vi "ElevShifter.vi"(5 "MaxPwr":dbl, 8 "Shift?":bool, 9 "PwrIn":dbl) -> (3 "PwrOut":dbl)   [LabVIEW 2017]
uses:
  <vilib>/Rock Robotics/WPI/Solenoid/Deprecated/WPI_SolenoidSetBool.vi
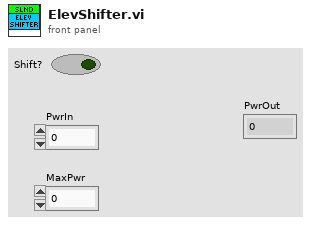
[diagram p1: front panel]
types:
  T1 = typedef "WPI_SolenoidDevRef.ctl" = cluster{"DevStatus":errorcluster, "Pneumatics Control Module":u8, "Forward Solenoid Channel":T2, "Reverse Solenoid Channel":T2}
  T2 = typedef "WPI_SolenoidChannel.ctl" = enum8{"Solenoid 0", "Solenoid 1", "Solenoid 2", "Solenoid 3", "Solenoid 4", "Solenoid 5", "Solenoid 6", "Solenoid 7", "Invalid"}
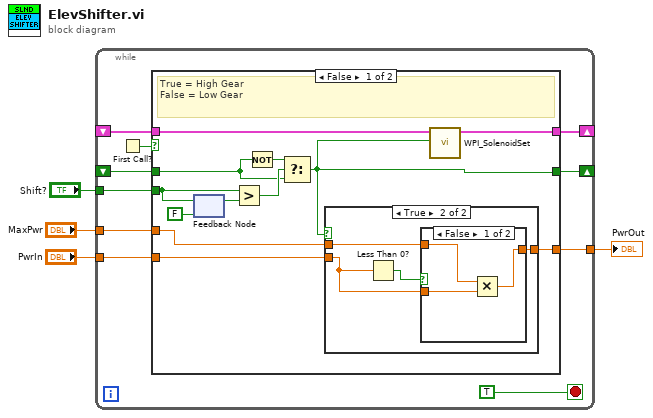
[diagram p0: block diagram]
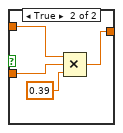
[diagram p3: hidden frame]
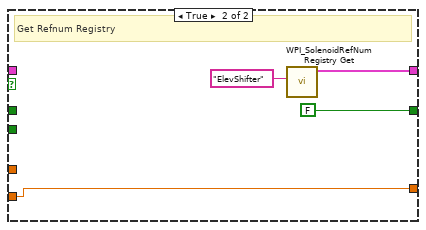
[diagram p4: hidden frame]
diagram:
  n1 = while {
    shift-right: [w13] -> _
    shift-left: _ -> [w12]
    tunnel: "Shift?" -> [w10]
    shift-right: [w9] -> _
    shift-left: _ -> [w8]
    tunnel: "MaxPwr" -> [w7]
    tunnel: "PwrIn" -> [w6]
    tunnel: [w5] -> w1
    stop <- TRUE stop-if-true
    n2 = First Call?() -> (First Call?: T/F=w11:bool)
    n3 = case shown="False" w11 {
      tunnel: [w20 w41] -> w13
      tunnel: w12 -> [w19 _]
      tunnel: w10 -> [w23 _]
      tunnel: [w15 FALSE] -> w9
      tunnel: w8 -> [w21 _]
      tunnel: w7 -> [w18 _]
      tunnel: w6 -> [w17 w39]
      tunnel: [w16 w39] -> w5
      frame False {
        # "True = High Gear\nFalse = Low Gear"
        n4 = feedback-in #1(w23) -> ()
        n5 = feedback #1(FALSE ("Shift?")) -> (w24:bool)
        n6 = Greater?(x=w23, y=w24) -> (0:w26:bool)
        n7 = Not(x=w21) -> (.not. x?=w25:bool)
        n8 = Select(t=w25, s=w26, f=w21) -> (s? t:f=w15:bool)
        n9 = case shown="True" w15 {
          tunnel: w18 -> [_ w30]
          tunnel: w17 -> [w27 w29]
          tunnel: [w27 w31] -> w16
          frame False {
          }
          frame True {
            n10 = Less Than 0?(x=w29) -> (x < 0?=w28:bool)
            n11 = case shown="False" w28 {
              tunnel: [w34 w35] -> w31
              tunnel: w30 -> [w33 w38]
              tunnel: w29 -> [w32 w37]
              frame False {
                n12 = Multiply(x=w33, y=w32) -> (x*y=w34:dbl)
              }
              frame True {
                n13 = Compound Arithmetic op=MULTIPLY(w38, w37, 0.39 ("value")) -> (w35:dbl)
              }
            }
          }
        }
        n14 = call-poly <vilib>:"WPI_SolenoidSet.vi"("Value"=w15, "SolenoidDevRef"=w19) -> ("SolenoidDevRef"=w20:T1)  [unwired: 8 in, 1 out]
      }
      frame True {
        # "Get Refnum Registry"
        n15 = call <vilib>:"WPI_SolenoidRefNum Registry Get.vi"("refnum name"="ElevShifter") -> ("SolenoidDevRef"=w41:T1)  [unwired: 9 in, 1 out]
      }
    }
  }
  "PwrOut" <- w1
